vi "0008H_DO_盐度补偿值写入.vi"(8 "error in (no error)":errorcluster caption="错误输入（无错误）", 10 "数值":sgl, 11 "MB session in":refnum<class "MB_Master.lvclass">) -> (0 "error out":errorcluster caption="错误输出", 3 "MB session out":refnum<class "MB_Master.lvclass">)   [LabVIEW 2016, in "斯坦道多参数.lvlib"]
uses:
  <vilib>/Plasmionique/MB Master/MB_Master/MB_Master.lvclass
  <vilib>/Plasmionique/MB Master/MB Master.lvlib
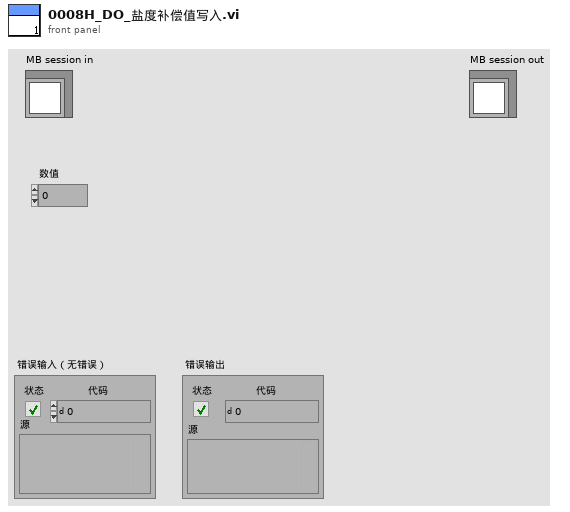
[diagram p1: front panel]
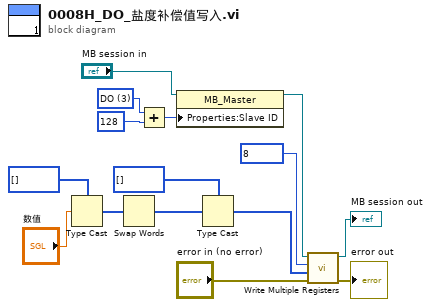
[diagram p0: block diagram]
diagram:
  w12 = u16 3 items=["NULL", "pH", "Cond", "DO", "Turb"] ("数值")
  n1 = Type Cast(type=u32[] [] ("数组 2"), x="数值") -> (*(type *) &x=w7:u32[])
  n2 = Swap Words(1:w7) -> (0:w5:u32[])
  n3 = Add(x=w12, y=u16 128) -> (x+y=w11:u16)
  n4 = property class="MB_Master"(reference="MB session in", "Properties:Slave ID"=w11) -> (reference out=w9:refnum<class "MB_Master.lvclass">)  [unwired: 1 in, 1 out]
  n5 = Type Cast(type=u16[] [] ("数组 2"), x=w5) -> (*(type *) &x=w3:u16[])
  n6 = call <vilib>:"Write Multiple Registers.vi"("error in (no error)"="error in (no error)", "values"=w3, "starting address"=u16 8, "MB session in"=w9) -> ("error out"=→"error out":errorcluster, "MB session out"=→"MB session out":refnum<class "MB_Master.lvclass">)  [unwired: 6 in]
